vi "BoundaryLimits.vi"(0 "UpperLimit":dbl, 1 "UpperValue":dbl, 2 "Input":dbl, 3 "LowerLimit":dbl, 4 "LowerValue":dbl) -> (5 "Output":dbl)   [LabVIEW 2014]
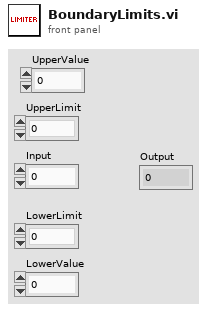
[diagram p1: front panel]
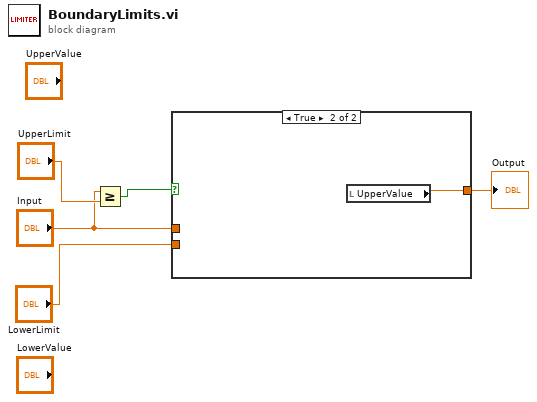
[diagram p0: block diagram]
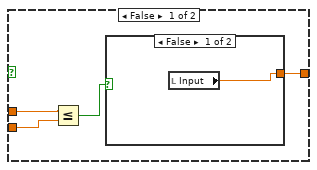
[diagram p2: hidden frame]
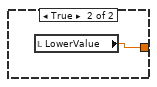
[diagram p3: hidden frame]
diagram:
  n1 = Greater Or Equal?(x="Input", y="UpperLimit") -> (x >= y?=w4:bool)
  n2 = case shown="True" w4 {
    tunnel: [w6 w12] -> w3
    tunnel: "Input" -> [w9 _]
    tunnel: "LowerLimit" -> [w8 _]
    frame False {
      n3 = Less Or Equal?(x=w9, y=w8) -> (x <= y?=w7:bool)
      n4 = case shown="False" w7 {
        tunnel: [w10 w11] -> w6
        frame False {
          n5 = local read "Input"() -> (w10:dbl)
        }
        frame True {
          n6 = local read "LowerValue"() -> (w11:dbl)
        }
      }
    }
    frame True {
      n7 = local read "UpperValue"() -> (w12:dbl)
    }
  }
  "Output" <- w3
